vi "Binary input.vi"() -> (3 "BIArray":u64)   [LabVIEW 2017]
uses:
  <vilib>/rvi/eio/common/nirviEmuTemplateMethod_errors.vi
  <vilib>/eio/EIONode/EIONode.xnode
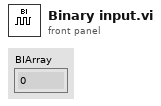
[diagram p1: front panel]
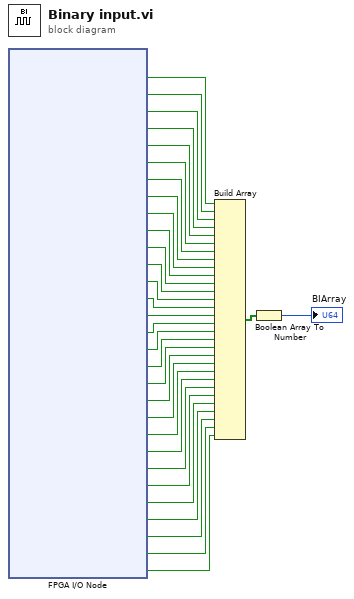
[diagram p0: block diagram]
diagram:
  n1 = xnode "FPGA I/O Node"() -> ("USER Push Button"=w32:bool, "Scan Clock"=w31:bool, "Mod2/DIO0"=w30:bool, "Mod2/DIO1"=w29:bool, "Mod2/DIO2"=w28:bool, "Mod2/DIO3"=w27:bool, "Mod3/DIO0"=w26:bool, "Mod3/DIO1"=w25:bool, "Mod3/DIO2"=w24:bool, "Mod3/DIO3"=w23:bool, "Mod3/DIO4"=w22:bool, "Mod3/DIO5"=w21:bool, "Mod3/DIO6"=w20:bool, "Mod3/DIO7"=w19:bool, "Mod4/DIO0"=w18:bool, "Mod4/DIO1"=w17:bool, "Mod4/DIO2"=w16:bool, "Mod4/DIO3"=w15:bool, "Mod4/DIO4"=w14:bool, "Mod4/DIO5"=w13:bool, "Mod4/DIO6"=w12:bool, "Mod4/DIO7"=w11:bool, "Mod5/DIO0"=w10:bool, "Mod5/DIO1"=w8:bool, "Mod5/DIO2"=w7:bool, "Mod5/DIO3"=w6:bool, "Mod5/DIO4"=w5:bool, "Mod5/DIO5"=w4:bool, "Mod5/DIO6"=w3:bool, "Mod5/DIO7"=w2:bool)  [unwired: 30 in, 30 out]
  n2 = Build Array(w32, w31, w30, w29, w28, w27, w26, w25, w24, w23, w22, w21, w20, w19, w18, w17, w16, w15, w14, w13, w12, w11, w10, w8, w7, w6, w5, w4, w3, w2) -> (w9:bool[])
  n3 = Boolean Array To Number(Boolean array=w9) -> (number=→"BIArray":u64)
